vi "Linear Ramp [U8].vi"(0 "Increment (1)":u8=1, 3 "# Elements":i32, 4 "Start (0)":u8) -> (5 "Ramp":u8[](array[numeric]))   [LabVIEW 2021, in "Arrays.lvlib"]
uses:
  Arrays.lvlib
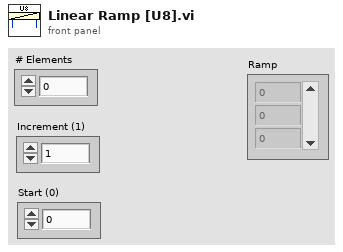
[diagram p1: front panel]
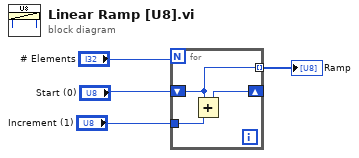
[diagram p0: block diagram]
diagram:
  n1 = for {
    N: "# Elements" -> [_]
    shift-right: [w6] -> _
    shift-left: "Start (0)" -> [w5]
    tunnel: "Increment (1)" -> [w7]
    tunnel: [w5] -> w1 mode=indexing
    n2 = Add(x=w5, y=w7) -> (x+y=w6:u8)
  }
  "Ramp" <- w1
